vi "createProcessCommandEvent.vi"(8 "error in (no error)":errorcluster, 11 "UserEvents in":refnum<class "UserEvents.lvclass">) -> (0 "error out":errorcluster, 3 "UserEvents out":refnum<class "UserEvents.lvclass">)   [LabVIEW 2016, in "UserEvents.lvclass"]
uses:
  UserEvents.lvclass
  Types/ProcessCommandEvent.ctl
  Commands/Command/Command.lvclass
  UserEvents.lvclass/UserEvents.ctl
  Types/M1M3SupportTypes.lvlib
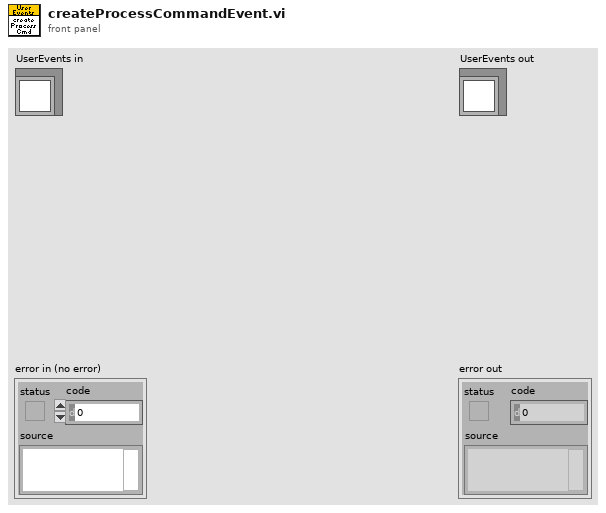
[diagram p1: front panel]
types:
  T1 = typedef "M1M3SupportTypes.lvlib/ProcessCommandEvent.ctl" = cluster{"Command":refnum<class "Command.lvclass">}
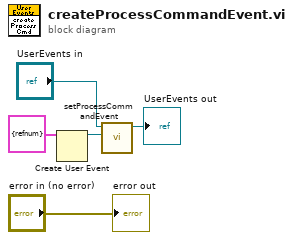
[diagram p0: block diagram]
diagram:
  n1 = Create User Event(user event datatype=T1 {"Command"=refnum} ("ProcessCommand")) -> (user event=w4:refnum<user-event>)  [unwired: 1 in, 1 out]
  n2 = call "setProcessCommandEvent.vi"("ProcessCommandEvent"=w4, "UserEvents in"="UserEvents in") -> ("UserEvents out"=→"UserEvents out":refnum<class "UserEvents.lvclass">)  [unwired: 9 in]
  "error out" <- "error in (no error)"
